vi "Close Instrument.vi"(8 "error in (no error)":errorcluster, 11 "Instrument.sample-registry":refnum<class "Instrument.sample-registry.lvclass">) -> (0 "error out":errorcluster, 3 "Instrument.sample-registry out":refnum<class "Instrument.sample-registry.lvclass">)   [LabVIEW 2019, in "Instrument.sample-registry.lvclass"]
uses:
  Instrument.sample-registry.lvclass
  <userlib>/LevyLab/Levylab Instruments/Instrument Types/VSource/Instrument.VSource.lvclass
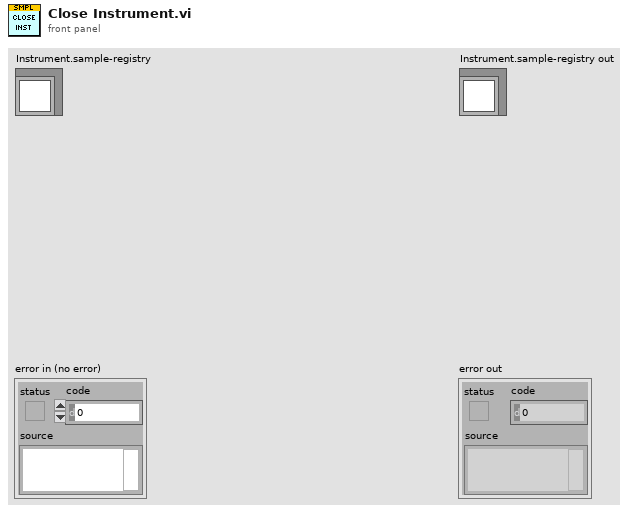
[diagram p1: front panel]
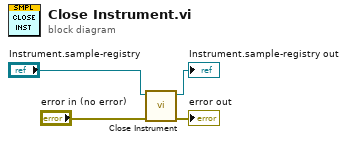
[diagram p0: block diagram]
diagram:
  n1 = call-parent "Close Instrument.vi"("error in (no error)"="error in (no error)", "Instrument in"="Instrument.sample-registry") -> ("error out"=→"error out":errorcluster, "Instrument out"=→"Instrument.sample-registry out":refnum<class "Instrument.sample-registry.lvclass">)  [unwired: 8 in]
